vi "Auto 3.vi"(8 "Error In":errorcluster) -> ()   [LabVIEW 2014]
uses:
  Robot Global Data.vi
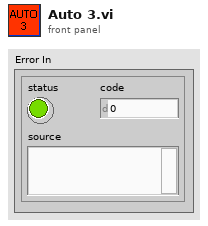
[diagram p1: front panel]
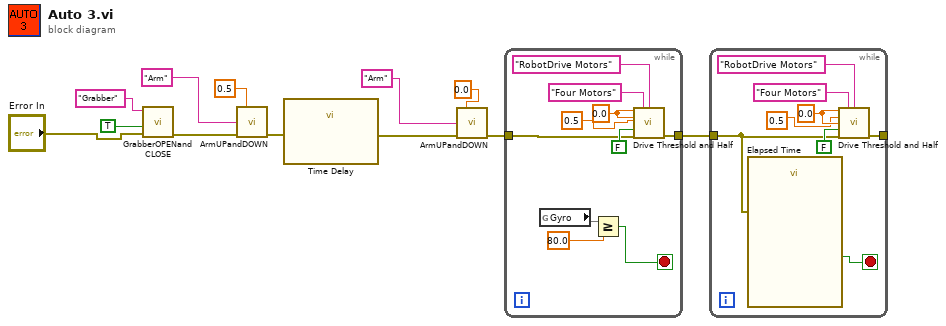
[diagram p0: block diagram]
diagram:
  n1 = call "GrabberOPENandCLOSE.vi"("Error In"="Error In", "Grabber Open/Close"=TRUE, "refnum name"="Grabber") -> ("Error Out"=w6:errorcluster)  [unwired: 8 in]
  n2 = call "ArmUPandDOWN.vi"("Arm Value"=0.5, "Arm"="Arm" ("refnum name"), "Error In"=w6) -> ("Error Out"=w8:errorcluster)  [unwired: 12 in]
  n3 = call "Time Delay"("error in (no error)"=w8) -> ("error out"=w11:errorcluster)  [unwired: 10 in]
  n4 = call "ArmUPandDOWN.vi"("Arm Value"=0.0, "Arm"="Arm" ("refnum name"), "Error In"=w11) -> ("Error Out"=w12:errorcluster)  [unwired: 12 in]
  n5 = while {
    tunnel: w12 -> [w19]
    tunnel: [w18] -> w1
    stop <- w13 stop-if-true
    w17 = 0.0 ("Arm Value")
    n6 = global read "Robot Global Data.vi" "Gyro"() -> (w15)
    n7 = Greater Or Equal?(x=w15, y=80.0) -> (x >= y?=w13:bool)
    n8 = call "Drive Threshold and Half.vi"("X In"=w17, "Drive refnum name"="Four Motors" ("refnum name"), "Send to DB Name"="RobotDrive Motors" ("Name"), "Y In"=w17, "R In"=0.5 ("X In"), "Speed Toggle"=FALSE ("Grabber Open/Close"), "Error In"=w19) -> ("Error Out"=w18:errorcluster)  [unwired: 8 in]
  }
  n9 = while {
    tunnel: w1 -> [w23]
    tunnel: [w27] -> _
    stop <- w24 stop-if-true
    w26 = 0.0 ("Arm Value")
    n10 = call "Elapsed Time"("error in (no error)"=w23) -> ("Time has Elapsed"=w24:bool)  [unwired: 11 in, 7 out]
    n11 = call "Drive Threshold and Half.vi"("X In"=w26, "Drive refnum name"="Four Motors" ("refnum name"), "Send to DB Name"="RobotDrive Motors" ("Name"), "Y In"=0.5 ("X In"), "R In"=w26, "Speed Toggle"=FALSE ("Grabber Open/Close"), "Error In"=w23) -> ("Error Out"=w27:errorcluster)  [unwired: 8 in]
  }
